vi "WVD Spectrogram.vi"(2 "time increment":i32=1 min=0, 3 "X":sgl[](array[numeric])) -> (0 "error":i32, 1 "WVD Spectrogram {X}":sgl[][](array[numeric]))   [LabVIEW 2017, in "NI_Gmath.lvlib"]
doc: "Computes the energy distribution of the input signal in the joint time-frequency domain using the Wigner-Ville distribution (WVD) algorithm."
uses:
  NI_Gmath.lvlib
  NI_AALPro.lvlib
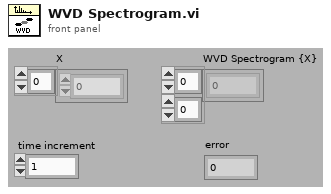
[diagram p1: front panel]
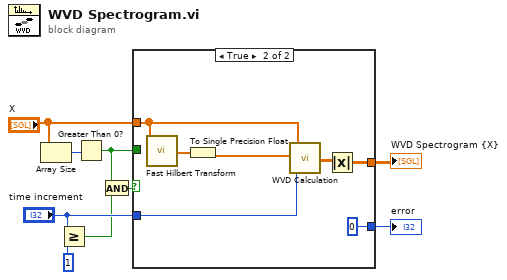
[diagram p0: block diagram]
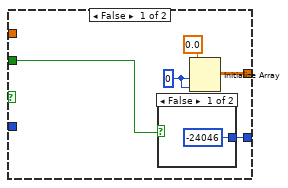
[diagram p2: hidden frame]
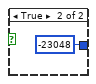
[diagram p3: hidden frame]
diagram:
  n1 = Array Size(array="X") -> (size(s)=w7:i32)
  n2 = Greater Or Equal?(x="time increment", y=1) -> (x >= y?=w4:bool)
  n3 = Greater Than 0?(x=w7) -> (x > 0?=w1:bool)
  n4 = And(x=w1, y=w4) -> (x .and. y?=w3:bool)
  n5 = case shown="True" w3 {
    tunnel: [w13 w22] -> w9
    tunnel: "X" -> [_ w20]
    tunnel: "time increment" -> [_ w19]
    tunnel: [w11 0] -> w8
    tunnel: w1 -> [w10 _]
    frame False {
      w12 = 0
      n6 = case shown="False" w10 {
        tunnel: [-24046 -23048] -> w11
        frame False {
        }
        frame True {
        }
      }
      n7 = Initialize Array(0.0, w12, w12) -> (w13:dbl[][])
    }
    frame True {
      n8 = call "Fast Hilbert Transform.vi"("X"=w20) -> ("Hilbert{X}"=w18:dbl[])  [unwired: 1 out]
      n9 = To Single Precision Float(number=w18) -> (single precision float=w23:sgl[])
      n10 = call "WVD Calculation.vi"("time increment"=w19, "H[s]"=w23, "s"=w20) -> ("Fourier[s(i-m)*g(m)]"=w21:sgl[][])
      n11 = Absolute Value(x=w21) -> (abs(x)=w22:sgl[][])
    }
  }
  "WVD Spectrogram {X}" <- w9
  "error" <- w8
